vi "Transmit.vi"(7 "packet? (f)":bool, 8 "error in (no error)":errorcluster, 10 "data":string, 11 "Socket.Base in":refnum<class "Socket.Base.lvclass">) -> (0 "error out":errorcluster, 2 "bytes written":i32, 3 "Socket.Base out":refnum<class "Socket.Base.lvclass">)   [LabVIEW 2014, in "Socket.lvlib" / "Socket.Base.lvclass"]
doc: "(Must be overridden.) Transmits the data, returns the number of bytes transmitted. See the individual child classes for the usage of the input parameters."
uses:
  Socket.Base.lvclass
  <vilib>/Utility/error.llb/Error Cluster From Error Code.vi
  <vilib>/ErrorRing/Error Ring.xnode
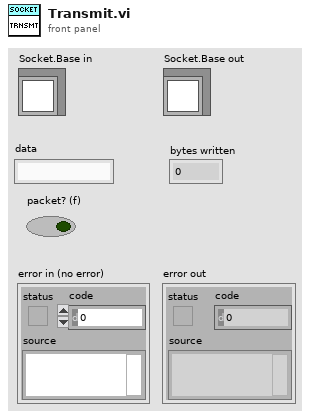
[diagram p1: front panel]
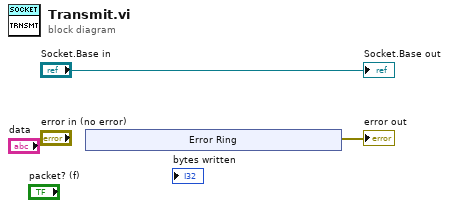
[diagram p0: block diagram]
diagram:
  n1 = xnode "Error Ring"() -> ("error out"=→"error out":errorcluster)
  "Socket.Base out" <- "Socket.Base in"
